vi "Handle Events.vi"(8 "error in (no error)":errorcluster, 11 "ListboxEventHandler":refnum<class "ListboxEventHandler.lvclass">) -> ()   [LabVIEW 2019, in "ActorEvents.lvlib" / "ListboxEventHandler.lvclass"]
uses:
  <vilib>/gpm_packages/@cs/mva-viewable/Source/ActorEvents/EventHandler/ListboxEventHandler/ListboxEventHandler.lvclass
  C:/Program Files/National Instruments/LabVIEW 2019/vi.lib/gpm_packages/@cs/mva-viewable/Source/ActorEvents/IEventHandler/IEventHandler.lvclass
  <vilib>/gpm_packages/@cs/mva-viewable/Source/ActorEvents/EventHandler/ListboxEventHandler/ListboxEventHandler.lvclass/ListboxEventHandler.ctl
  <vilib>/gpm_packages/@cs/mva-viewable/Source/ActorEvents/IEventHandler/IEventHandler.lvclass/IEventHandler.ctl
  <vilib>/ActorFramework/Message Enqueuer/Message Enqueuer.lvclass/Message Enqueuer.ctl
  <vilib>/event_ctls.llb/lveventtype.ctl
  <vilib>/gpm_packages/@cs/mva-viewable/Source/ActorEvents/IEventAggregator Messages/EventDataMessage/EventDataMessage.lvclass/EventDataMessage.ctl
  <vilib>/Utility/miscctls.llb/LVRowAndColumnTypeDef.ctl
  <vilib>/gpm_packages/@cs/mva-viewable/Source/ActorEvents/IEventAggregator Messages/ListboxEditCellMsg/ListboxEditCellMsg.lvclass/ListboxEditCellMsg.ctl
  <vilib>/gpm_packages/@cs/mva-viewable/Source/ActorEvents/IEventAggregator Messages/ControlKeyDownMsg/ControlKeyDownMsg.lvclass/ControlKeyDownMsg.ctl
  <vilib>/gpm_packages/@cs/mva-viewable/Source/ActorEvents/IEventAggregator Messages/ControlMouseDownMsg/ControlMouseDownMsg.lvclass/ControlMouseDownMsg.ctl
  <vilib>/gpm_packages/@cs/mva-viewable/Source/ActorEvents/IEventAggregator Messages/ControlDragStartingMsg/ControlDragStartingMsg.lvclass/ControlDragStartingMsg.ctl
  <vilib>/gpm_packages/@cs/mva-viewable/Source/ActorEvents/IEventAggregator Messages/ControlDragSourceUpdateMsg/ControlDragSourceUpdateMsg.lvclass/ControlDragSourceUpdateMsg.ctl
  <vilib>/gpm_packages/@cs/mva-viewable/Source/ActorEvents/IEventAggregator Messages/EventDataMessage/Read Discarded.vi
  <vilib>/gpm_packages/@cs/mva-viewable/Source/ActorEvents/IEventAggregator Messages/ListboxEditCellMsg/Accessors/Read String.vi
  <vilib>/gpm_packages/@cs/mva-viewable/Source/ActorEvents/IEventAggregator Messages/ControlKeyDownMsg/Accessors/Read Char.vi
  <vilib>/gpm_packages/@cs/mva-viewable/Source/ActorEvents/IEventAggregator Messages/ControlKeyDownMsg/Accessors/Read VKey.vi
  <vilib>/gpm_packages/@cs/mva-viewable/Source/ActorEvents/IEventAggregator Messages/ControlKeyDownMsg/Accessors/Read Mods.vi
  <vilib>/gpm_packages/@cs/mva-viewable/Source/ActorEvents/IEventAggregator Messages/ControlKeyDownMsg/Accessors/Read PlatMods.vi
  <vilib>/gpm_packages/@cs/mva-viewable/Source/ActorEvents/IEventAggregator Messages/ControlKeyDownMsg/Accessors/Read FocusObj.vi
  <vilib>/gpm_packages/@cs/mva-viewable/Source/ActorEvents/IEventAggregator Messages/ControlMouseDownMsg/Accessors/Read Button.vi
  <vilib>/gpm_packages/@cs/mva-viewable/Source/ActorEvents/IEventAggregator Messages/ControlMouseDownMsg/Accessors/Read Mods.vi
  <vilib>/gpm_packages/@cs/mva-viewable/Source/ActorEvents/IEventAggregator Messages/ControlMouseDownMsg/Accessors/Read PlatMods.vi
  <vilib>/gpm_packages/@cs/mva-viewable/Source/ActorEvents/IEventAggregator Messages/ControlDragStartingMsg/Accessors/Read Data.vi
  <vilib>/gpm_packages/@cs/mva-viewable/Source/ActorEvents/IEventAggregator Messages/ControlDragStartingMsg/Accessors/Read Drag Mode.vi
  <vilib>/gpm_packages/@cs/mva-viewable/Source/ActorEvents/IEventAggregator Messages/ControlDragSourceUpdateMsg/Accessors/Read Cursor.vi
  <vilib>/gpm_packages/@cs/mva-viewable/Source/ActorEvents/IEventHandler/Accessors/Read Timeout [ms].vi
  <vilib>/gpm_packages/@cs/mva-viewable/Source/ActorEvents/IEventHandler/Accessors/Read Event Filter.vi
  <vilib>/gpm_packages/@cs/mva-viewable/Source/ActorEvents/IEventHandler/Accessors/Read EventAggregator Enqueuer.vi
  <vilib>/gpm_packages/@cs/mva-viewable/Source/ActorEvents/IEventHandler/Accessors/Read Timeout Message.vi
  <vilib>/gpm_packages/@cs/mva-viewable/Source/ActorEvents/IEventHandler/Accessors/Read Timeout Message Priority.vi
  <vilib>/gpm_packages/@cs/mva-viewable/Source/ActorEvents/IEventAggregator Messages/ShortcutMenuSelectionMsg/ShortcutMenuSelectionMsg.lvclass
  C:/Program Files/National Instruments/LabVIEW 2019/vi.lib/gpm_packages/@cs/mva-viewable/Source/ActorEvents/IEventAggregator Messages/EventDataMessage/EventDataMessage.lvclass
  <vilib>/gpm_packages/@cs/mva-viewable/Source/ActorEvents/IEventAggregator Messages/ShortcutMenuActivationMsg/ShortcutMenuActivationMsg.lvclass
  <vilib>/gpm_packages/@cs/mva-viewable/Source/ActorEvents/IEventAggregator Messages/ListboxEditCellMsg/ListboxEditCellMsg.lvclass
  <vilib>/gpm_packages/@cs/mva-viewable/Source/ActorEvents/IEventAggregator Messages/ControlKeyDownMsg/ControlKeyDownMsg.lvclass
  <vilib>/gpm_packages/@cs/mva-viewable/Source/ActorEvents/IEventAggregator Messages/ControlMouseDownMsg/ControlMouseDownMsg.lvclass
  <vilib>/gpm_packages/@cs/mva-viewable/Source/ActorEvents/IEventAggregator Messages/ControlDropMsg/ControlDropMsg.lvclass
  <vilib>/gpm_packages/@cs/mva-viewable/Source/ActorEvents/IEventAggregator Messages/ControlDragOverMsg/ControlDragOverMsg.lvclass
  <vilib>/gpm_packages/@cs/mva-viewable/Source/ActorEvents/IEventAggregator Messages/ControlDragStartingMsg/ControlDragStartingMsg.lvclass
  <vilib>/gpm_packages/@cs/mva-viewable/Source/ActorEvents/IEventAggregator Messages/ControlDragSourceUpdateMsg/ControlDragSourceUpdateMsg.lvclass
  <vilib>/ActorFramework/Message Priority Queue/Priority Enqueue.vi
  <vilib>/gpm_packages/@cs/mva-viewable/Source/ActorEvents/IEventFilter/IEventFilter.lvclass
  <vilib>/ActorFramework/Message Enqueuer/Message Enqueuer.lvclass
  <vilib>/ActorFramework/Message/Message.lvclass
  <vilib>/gpm_packages/@cs/mva-viewable/Source/ActorEvents/IEventAggregator Messages/ValueChangeMsg/ValueChangeMsg.lvclass
  <vilib>/gpm_packages/@cs/mva-viewable/Source/ActorEvents/IEventAggregator Messages/ControlMouseUpMsg/ControlMouseUpMsg.lvclass
  <vilib>/gpm_packages/@cs/mva-viewable/Source/ActorEvents/IEventAggregator Messages/ListboxDoubleClickMsg/ListboxDoubleClickMsg.lvclass
  <vilib>/gpm_packages/@cs/mva-viewable/Source/ActorEvents/IEventAggregator Messages/ControlMouseEnterMsg/ControlMouseEnterMsg.lvclass
  <vilib>/gpm_packages/@cs/mva-viewable/Source/ActorEvents/IEventAggregator Messages/ControlMouseLeaveMsg/ControlMouseLeaveMsg.lvclass
  <vilib>/gpm_packages/@cs/mva-viewable/Source/ActorEvents/IEventAggregator Messages/ControlKeyUpMsg/ControlKeyUpMsg.lvclass
  <vilib>/gpm_packages/@cs/mva-viewable/Source/ActorEvents/IEventAggregator Messages/ControlDragEndedMsg/ControlDragEndedMsg.lvclass
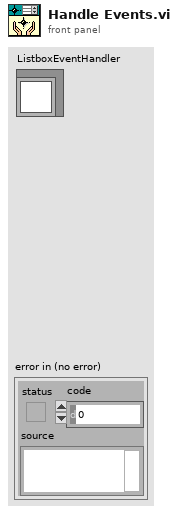
[diagram p1: front panel]
types:
  T1 = typedef "ActorEvents.lvlib/IEventFilter.lvclass/EventFilter Reference.ctl" = refnum<data-value>
  T2 = typedef "Actor Framework.lvlib/Message Enqueuer.lvclass/Message Priority.ctl" = enum16{"Low", "Normal", "High"}
  T3 = typedef "lveventtype.ctl" = enum32{"Null", "Timeout", "Annotation Menu Selection", "Annotation Menu Selection?", "App Instance Close", "App Instance Close?", "Autoscale Range Change", "Bookmark Info Change", "Cell Edit", "Cell Edit?", "Cursor Grab", "Cursor Grab?", "Cursor Menu Selection", "Cursor Menu Selection?", "Cursor Move", "Cursor Release", "Data Change", "Direction Change", "Display State Change", "Drag Ended", "Drag Enter", "Drag Leave", "Drag Over", "Drag Source Update", "Drag Starting", "Drag Starting?", "Drop", "Exec State Change", "Key Down", "Key Down?", "Key Repeat", "Key Repeat?", "Key Up", "Listbox Double Click", "Menu Activation?", "Menu Selection (App)", "Menu Selection? (App)", "Menu Selection (User)", "Mouse Down", "Mouse Down?", "Mouse Enter", "Mouse Leave", "Mouse Move", "Mouse Up", "Mouse Wheel", "NI Security User Change (App)", "Pane Size", "Panel Close", "Panel Close?", "Panel Resize", "Plot Attribute Change", "Scale Range Change", "Shortcut Menu Activation?", "Shortcut Menu Selection (App)", "Shortcut Menu Selection? (App)", "Shortcut Menu Selection (User)", "Tree Double Click", "Tree Drag", "Tree Drag?", "Tree Drop", "Tree Drop?", "Tree Item Close", "Tree Item Close?", "Tree Item Open", "Tree Item Open?", "User Event", "Value Change"}
  T4 = typedef "LVRowAndColumnTypeDef.ctl" = cluster{"Row":i32, "Column":i32}
  T5 = typedef "LVPoint32TypeDef.ctl" = cluster{"Horizontal":i32, "Vertical":i32}
  T6 = cluster{"Shift":bool, "Ctrl":bool, "Alt":bool, "Cmd":bool, "Opt":bool}
  T7 = typedef "eventvkey.ctl" = enum16{"ASCII", "Enter", "Return", "Shift", "Ctrl", "Alt", "Cmd", "Opt", "Caps", "NumLock", "Clear", "Break", "Up", "Down", "Left", "Right", "Insert", "Delete", "Home", "End", "PageUp", "PageDown", "Escape", "Help", "Pause", "ScrollLock", "F1", "F2", "F3", "F4", "F5", "F6", "F7", "F8", "F9", "F10", "F11", "F12", "F13", "F14", "F15", "F16", "F17", "F18", "F19", "F20", "F21", "F22", "F23", "F24", "Play", "VolumeUp", "VolumeDown", "Mute", "Two Byte Char"}
  T8 = cluster{"data name":string, "drag data":variant}[]
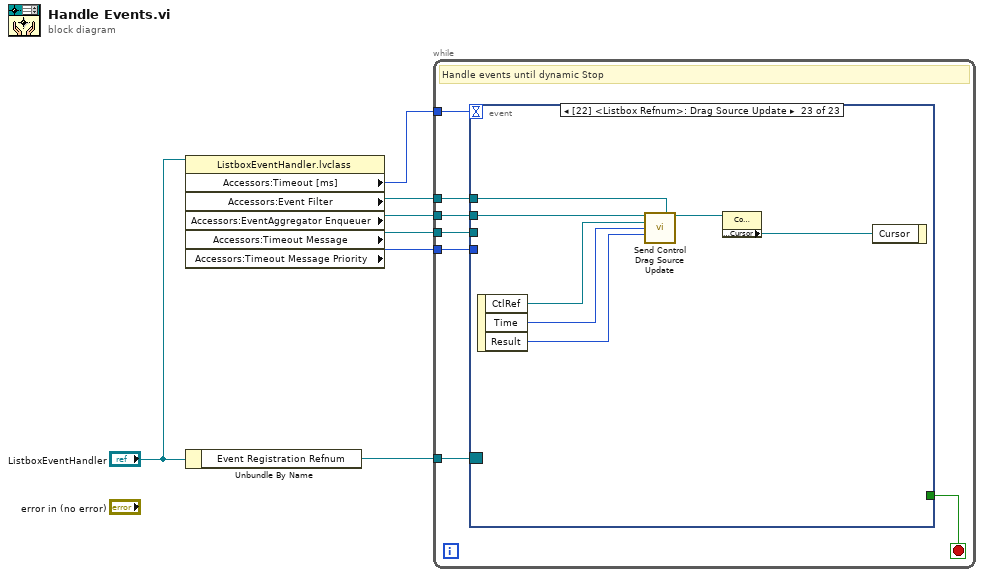
[diagram p0: block diagram]
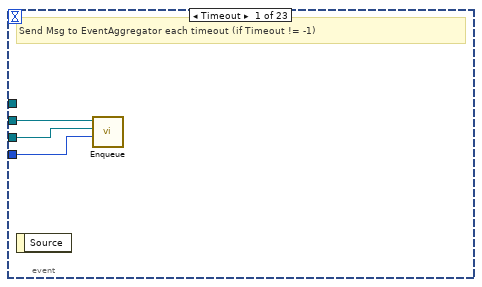
[diagram p2: hidden frame]
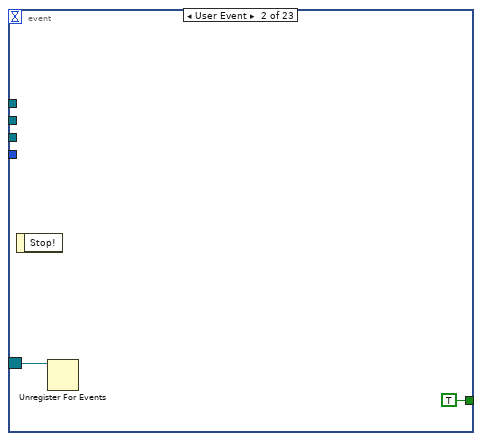
[diagram p3: hidden frame]
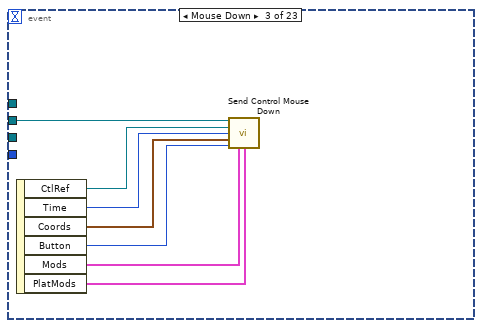
[diagram p4: hidden frame]
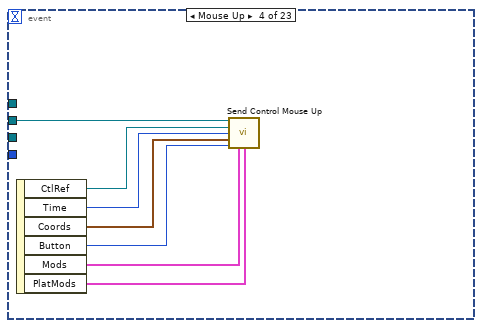
[diagram p5: hidden frame]
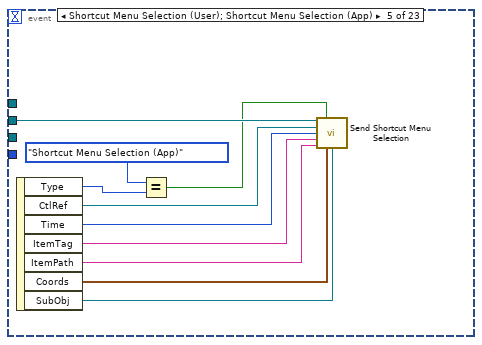
[diagram p6: hidden frame]
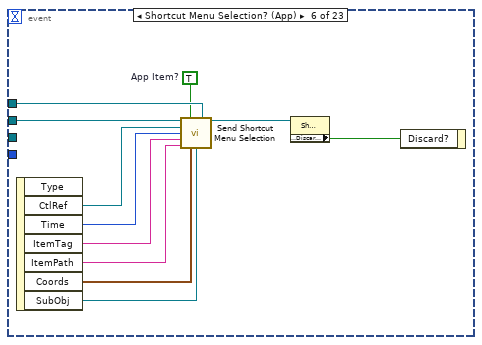
[diagram p7: hidden frame]
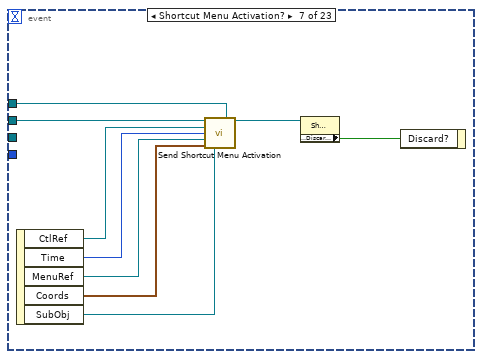
[diagram p8: hidden frame]
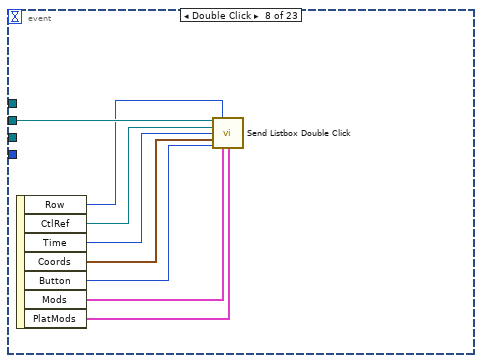
[diagram p9: hidden frame]
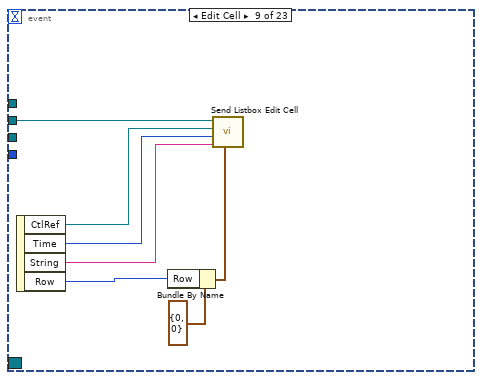
[diagram p10: hidden frame]
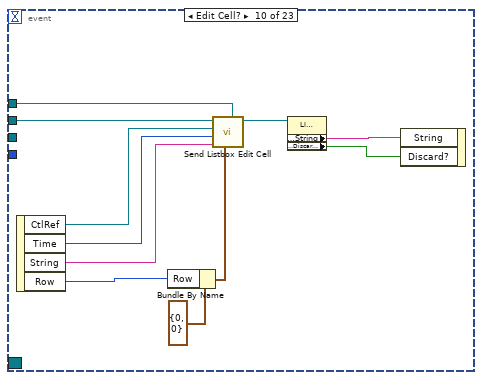
[diagram p11: hidden frame]
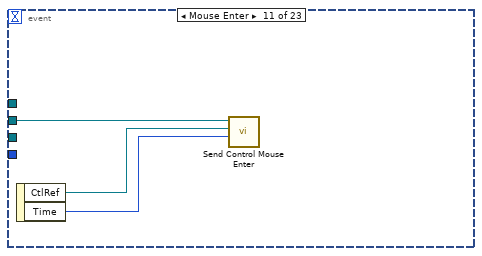
[diagram p12: hidden frame]
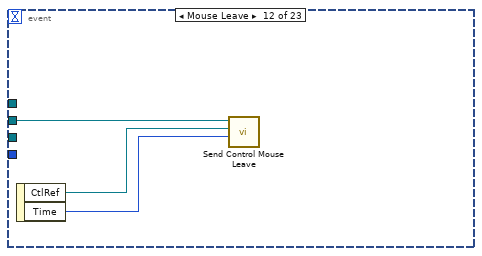
[diagram p13: hidden frame]
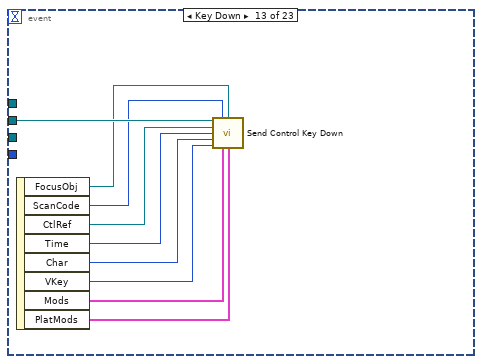
[diagram p14: hidden frame]
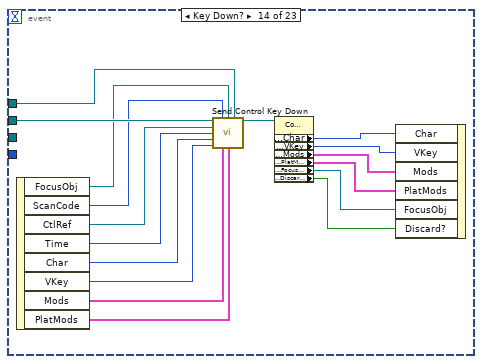
[diagram p15: hidden frame]
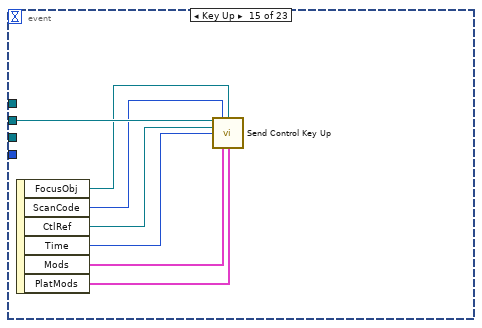
[diagram p16: hidden frame]
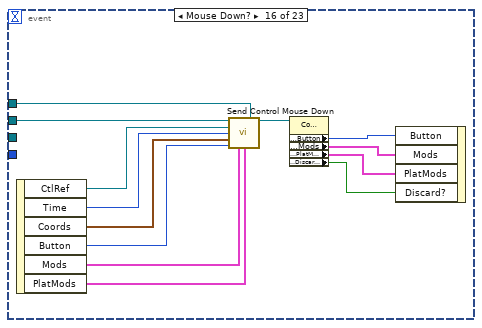
[diagram p17: hidden frame]
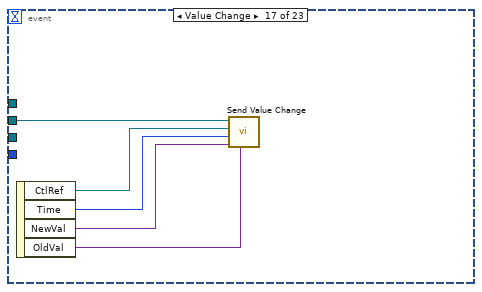
[diagram p18: hidden frame]
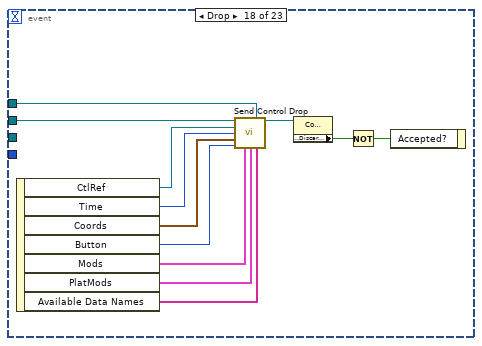
[diagram p19: hidden frame]
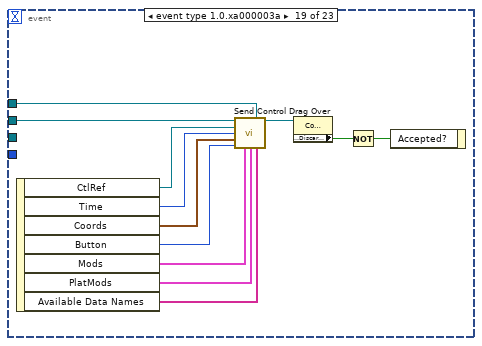
[diagram p20: hidden frame]
diagram:
  n1 = property class="ListboxEventHandler.lvclass"(reference="ListboxEventHandler") -> ("Accessors:Timeout [ms]"=w5:i32, "Accessors:Event Filter"=w3:T1, "Accessors:EventAggregator Enqueuer"=w4:refnum<class "Message Enqueuer.lvclass">, "Accessors:Timeout Message"=w2:refnum<class "Message.lvclass">, "Accessors:Timeout Message Priority"=w1:T2)  [unwired: 1 in, 2 out]
  n2 = Unbundle By Name("ListboxEventHandler") -> ("Event Registration Refnum"=w7:refnum<event-registration>)
  n3 = while {
    tunnel: w7 -> [w14]
    tunnel: w4 -> [w13]
    tunnel: w2 -> [w12]
    tunnel: w1 -> [w11]
    tunnel: w5 -> [w10]
    tunnel: w3 -> [w8]
    stop <- w9 stop-if-true
    # "Handle events until dynamic Stop"
    n4 = event shown="[22] <Listbox Refnum>: Drag Source Update" {
      selector: w14 -> [_ w19 _ _ _ _ _ _ _ _ _ _ _ _ _ _ _ _ _ _ _ _ _]
      dyn-events: _ -> [_ _ _ _ _ _ _ _ _ _ _ _ _ _ _ _ _ _ _ _ _ _ _]
      timeout: w10 -> [_ _ _ _ _ _ _ _ _ _ _ _ _ _ _ _ _ _ _ _ _ _ _]
      tunnel: [_ TRUE ("Stop!") _ _ _ _ _ _ _ _ _ _ _ _ _ _ _ _ _ _ _ _ _] -> w9
      tunnel: w13 -> [w17 _ w26 w33 w43 w54 w63 w71 w78 w89 w92 w95 w104 w121 w128 w141 w146 w156 w168 w174 w183 w197 w204]
      tunnel: w12 -> [w16 _ _ _ _ _ _ _ _ _ _ _ _ _ _ _ _ _ _ _ _ _ _]
      tunnel: w11 -> [w15 _ _ _ _ _ _ _ _ _ _ _ _ _ _ _ _ _ _ _ _ _ _]
      tunnel: w8 -> [_ _ _ _ _ w47 w57 _ _ w82 _ _ _ w111 _ w134 _ w147 w159 _ _ w187 w203]
      event Timeout {
        # "Send Msg to EventAggregator each timeout (if Timeout != -1)"
        n5 = event-data() -> ()  [unwired: 1 in, 1 out]
        n6 = call <vilib>:"Enqueue.vi"("Message Priority (Normal)"=w15, "Message"=w16, "Message Enqueuer in"=w17) -> ()  [unwired: 7 in, 2 out]
      }
      event User Event {
        n7 = event-data() -> ()  [unwired: 1 in, 1 out]
        n8 = Unregister For Events(event registration refnum=w19) -> ()  [unwired: 1 in, 1 out]
      }
      event Mouse Down {
        n9 = event-data() -> ("CtlRef"=w25:refnum<vi>, "Time"=w24:u32, "Coords"=w23:T5, "Button"=w22:u16, "Mods"=w21:cluster{"Double Click":bool, "Menu Key":bool}, "PlatMods"=w20:T6)  [unwired: 1 in]
        n10 = call <vilib>:"Send Control Mouse Down.vi"("Message Enqueuer in"=w26, "Ctl Refnum"=w25, "Time"=w24, "Coords"=w23, "Button"=w22, "Mods"=w21, "PlatMods"=w20) -> ()  [unwired: 7 in, 2 out]
      }
      event Mouse Up {
        n11 = event-data() -> ("CtlRef"=w32:refnum<vi>, "Time"=w31:u32, "Coords"=w30:T5, "Button"=w29:u16, "Mods"=w28:cluster{"Double Click":bool, "Menu Key":bool}, "PlatMods"=w27:T6)  [unwired: 1 in]
        n12 = call <vilib>:"Send Control Mouse Up.vi"("Message Enqueuer in"=w33, "Ctl Refnum"=w32, "Time"=w31, "Coords"=w30, "Button"=w29, "Mods"=w28, "PlatMods"=w27) -> ()  [unwired: 8 in, 1 out]
      }
      event Shortcut Menu Selection (User); Shortcut Menu Selection (App) {
        n13 = event-data() -> ("Type"=w36:T3, "CtlRef"=w42:refnum<vi>, "Time"=w41:u32, "ItemTag"=w40:string, "ItemPath"=w39:string, "Coords"=w38:T5, "SubObj"=w37:refnum<vi>)  [unwired: 1 in]
        n14 = Equal?(x=lveventtype."Shortcut Menu Selection (App)", y=w36) -> (x = y?=w35:bool)
        n15 = call <vilib>:"Send Shortcut Menu Selection.vi"("Message Enqueuer in"=w43, "App Item?"=w35, "CtlRef"=w42, "Time"=w41, "Item Tag"=w40, "Item Path"=w39, "Coords"=w38, "SubObj"=w37) -> ()  [unwired: 6 in, 2 out]
      }
      event Shortcut Menu Selection? (App) {
        w46 = TRUE  # App Item?
        n16 = event-data() -> ("CtlRef"=w53:refnum<vi>, "Time"=w52:u32, "ItemTag"=w51:string, "ItemPath"=w50:string, "Coords"=w49:T5, "SubObj"=w48:refnum<vi>)  [unwired: 1 in, 1 out]
        n17 = call <vilib>:"Send Shortcut Menu Selection.vi"("Message Enqueuer in"=w54, "App Item?"=w46, "EventFilter Reference"=w47, "CtlRef"=w53, "Time"=w52, "Item Tag"=w51, "Item Path"=w50, "Coords"=w49, "SubObj"=w48) -> ("Filtered EventDataMessage"=w45:refnum<class "ShortcutMenuSelectionMsg.lvclass">)  [unwired: 5 in, 1 out]
        n18 = property class="ShortcutMenuSelectionMsg.lvclas"(reference=w45) -> ("Accessors:Discarded?"=w44:bool)  [unwired: 1 in, 2 out]
        n19 = event-data("Discard?"=w44) -> ()  [unwired: 1 in, 1 out]
      }
      event Shortcut Menu Activation? {
        n20 = event-data() -> ("CtlRef"=w58:refnum<vi>, "Time"=w62:u32, "MenuRef"=w59:refnum<k9>, "Coords"=w61:T5, "SubObj"=w60:refnum<vi>)  [unwired: 1 in]
        n21 = call <vilib>:"Send Shortcut Menu Activation.vi"("Message Enqueuer in"=w63, "EventFilter Reference"=w57, "CtlRef"=w58, "Time"=w62, "MenuRef"=w59, "Coords"=w61, "SubObj"=w60) -> ("Filtered EventDataMessage"=w56:refnum<class "ShortcutMenuActivationMsg.lvclass">)  [unwired: 7 in, 1 out]
        n22 = property class="ShortcutMenuActivationMsg.lvcla"(reference=w56) -> ("Accessors:Discarded?"=w55:bool)  [unwired: 1 in, 2 out]
        n23 = event-data("Discard?"=w55) -> ()  [unwired: 1 in, 1 out]
      }
      event Double Click {
        n24 = event-data() -> ("Row"=w64:i32, "CtlRef"=w70:refnum<vi>, "Time"=w69:u32, "Coords"=w68:T5, "Button"=w67:u16, "Mods"=w66:cluster{"Double Click":bool, "Menu Key":bool}, "PlatMods"=w65:T6)  [unwired: 1 in]
        n25 = call <vilib>:"Send Listbox Double Click.vi"("Message Enqueuer in"=w71, "Row"=w64, "Ctl Refnum"=w70, "Time"=w69, "Coords"=w68, "Button"=w67, "Mods"=w66, "PlatMods"=w65) -> ()  [unwired: 7 in, 1 out]
      }
      event Edit Cell {
        n26 = event-data() -> ("CtlRef"=w77:refnum<vi>, "Time"=w76:u32, "String"=w75:string, "Row"=w74:i32)  [unwired: 1 in]
        n27 = Bundle By Name(cluster=T4 {"Row"=0, "Column"=0} ("Coords"), "Row"=w74) -> (w72:T4)
        n28 = call <vilib>:"Send Listbox Edit Cell.vi"("Coords"=w72, "String"=w75, "Time"=w76, "CtlRef"=w77, "Message Enqueuer in"=w78) -> ()  [unwired: 5 in, 2 out]
      }
      event Edit Cell? {
        n29 = event-data() -> ("CtlRef"=w88:refnum<vi>, "Time"=w87:u32, "String"=w86:string, "Row"=w85:i32)  [unwired: 1 in]
        n30 = Bundle By Name(cluster=T4 {"Row"=0, "Column"=0} ("Coords"), "Row"=w85) -> (w83:T4)
        n31 = call <vilib>:"Send Listbox Edit Cell.vi"("EventFilter Reference"=w82, "Coords"=w83, "String"=w86, "Time"=w87, "CtlRef"=w88, "Message Enqueuer in"=w89) -> ("Filtered EventDataMessage"=w81:refnum<class "ListboxEditCellMsg.lvclass">)  [unwired: 4 in, 1 out]
        n32 = property class="ListboxEditCellMsg.lvclass"(reference=w81) -> ("Accessors:String"=w80:string, "Accessors:Discarded?"=w79:bool)  [unwired: 1 in, 2 out]
        n33 = event-data("String"=w80, "Discard?"=w79) -> ()  [unwired: 1 in, 1 out]
      }
      event Mouse Enter {
        n34 = event-data() -> ("CtlRef"=w91:refnum<vi>, "Time"=w90:u32)  [unwired: 1 in]
        n35 = call <vilib>:"Send Control Mouse Enter.vi"("Time"=w90, "Ctl Refnum"=w91, "Message Enqueuer in"=w92) -> ()  [unwired: 8 in, 1 out]
      }
      event Mouse Leave {
        n36 = event-data() -> ("CtlRef"=w94:refnum<vi>, "Time"=w93:u32)  [unwired: 1 in]
        n37 = call <vilib>:"Send Control Mouse Leave.vi"("Time"=w93, "Ctl Refnum"=w94, "Message Enqueuer in"=w95) -> ()  [unwired: 8 in, 1 out]
      }
      event Key Down {
        n38 = event-data() -> ("FocusObj"=w103:refnum<vi>, "ScanCode"=w102:i16, "CtlRef"=w101:refnum<vi>, "Time"=w100:u32, "Char"=w99:i16, "VKey"=w98:T7, "Mods"=w97:cluster{"Num Pad":bool, "Menu Key":bool}, "PlatMods"=w96:T6)  [unwired: 1 in]
        n39 = call <vilib>:"Send Control Key Down.vi"("Message Enqueuer in"=w104, "ScanCode"=w102, "FocusObj"=w103, "CtlRef"=w101, "Time"=w100, "Char"=w99, "VKey"=w98, "Mods"=w97, "PlatMods"=w96) -> ()  [unwired: 5 in, 2 out]
      }
      event Key Down? {
        n40 = event-data() -> ("FocusObj"=w120:refnum<vi>, "ScanCode"=w119:i16, "CtlRef"=w118:refnum<vi>, "Time"=w117:u32, "Char"=w116:i16, "VKey"=w115:T7, "Mods"=w114:cluster{"Num Pad":bool, "Menu Key":bool}, "PlatMods"=w113:T6)  [unwired: 1 in]
        n41 = call <vilib>:"Send Control Key Down.vi"("Message Enqueuer in"=w121, "ScanCode"=w119, "FocusObj"=w120, "EventFilter Reference"=w111, "CtlRef"=w118, "Time"=w117, "Char"=w116, "VKey"=w115, "Mods"=w114, "PlatMods"=w113) -> ("Filtered EventDataMessage"=w112:refnum<class "ControlKeyDownMsg.lvclass">)  [unwired: 4 in, 1 out]
        n42 = property class="ControlKeyDownMsg.lvclass"(reference=w112) -> ("Accessors:Char"=w110:i16, "Accessors:VKey"=w109:T7, "Accessors:Mods"=w108:cluster{"Double Click":bool, "Menu Key":bool}, "Accessors:PlatMods"=w107:T6, "Accessors:FocusObj"=w106:refnum<vi>, "Accessors:Discarded?"=w105:bool)  [unwired: 1 in, 2 out]
        n43 = event-data("Char"=w110, "VKey"=w109, "Mods"=w108, "PlatMods"=w107, "FocusObj"=w106, "Discard?"=w105) -> ()  [unwired: 1 in, 1 out]
      }
      event Key Up {
        n44 = event-data() -> ("FocusObj"=w127:refnum<vi>, "ScanCode"=w126:i16, "CtlRef"=w125:refnum<vi>, "Time"=w124:u32, "Mods"=w123:cluster{"Num Pad":bool, "Menu Key":bool}, "PlatMods"=w122:T6)  [unwired: 1 in]
        n45 = call <vilib>:"Send Control Key Up.vi"("Message Enqueuer in"=w128, "ScanCode"=w126, "FocusObj"=w127, "Ctl Refnum"=w125, "Time"=w124, "Mods"=w123, "PlatMods"=w122) -> ()  [unwired: 8 in, 1 out]
      }
      event Mouse Down? {
        n46 = event-data() -> ("CtlRef"=w140:refnum<vi>, "Time"=w139:u32, "Coords"=w138:T5, "Button"=w137:u16, "Mods"=w136:cluster{"Double Click":bool, "Menu Key":bool}, "PlatMods"=w135:T6)  [unwired: 1 in]
        n47 = call <vilib>:"Send Control Mouse Down.vi"("Message Enqueuer in"=w141, "EventFilter Reference"=w134, "Ctl Refnum"=w140, "Time"=w139, "Coords"=w138, "Button"=w137, "Mods"=w136, "PlatMods"=w135) -> ("Filtered EventDataMessage"=w133:refnum<class "ControlMouseDownMsg.lvclass">)  [unwired: 6 in, 1 out]
        n48 = property class="ControlMouseDownMsg.lvclass"(reference=w133) -> ("Accessors:Button"=w132:u16, "Accessors:Mods"=w131:cluster{"Double Click":bool, "Menu Key":bool}, "Accessors:PlatMods"=w130:T6, "Accessors:Discarded?"=w129:bool)  [unwired: 1 in, 2 out]
        n49 = event-data("Button"=w132, "Mods"=w131, "PlatMods"=w130, "Discard?"=w129) -> ()  [unwired: 1 in, 1 out]
      }
      event Value Change {
        n50 = event-data() -> ("CtlRef"=w143:refnum<vi>, "Time"=w145:u32, "NewVal"=w144:variant, "OldVal"=w142:variant)  [unwired: 1 in]
        n51 = call <vilib>:"Send Value Change.vi"("Old Value"=w142, "New Value"=w144, "Time"=w145, "Ctl Refnum"=w143, "Message Enqueuer in"=w146) -> ()  [unwired: 6 in, 1 out]
      }
      event Drop {
        n52 = event-data() -> ("CtlRef"=w154:refnum<vi>, "Time"=w153:u32, "Coords"=w152:T5, "Button"=w151:u16, "Mods"=w150:cluster{"Double Click":bool, "Menu Key":bool}, "PlatMods"=w149:T6, "Available Data Names"=w148:string[])  [unwired: 1 in]
        n53 = call <vilib>:"Send Control Drop.vi"("Message Enqueuer in"=w156, "EventFilter Reference"=w147, "CtlRef"=w154, "Time"=w153, "Coords"=w152, "Button"=w151, "Mods"=w150, "PlatMods"=w149, "Available Data Names"=w148) -> ("Filtered EventDataMessage"=w157:refnum<class "ControlDropMsg.lvclass">)  [unwired: 5 in, 1 out]
        n54 = property class="ControlDropMsg.lvclass"(reference=w157) -> ("Accessors:Discarded?"=w158:bool)  [unwired: 1 in, 2 out]
        n55 = Not(x=w158) -> (.not. x?=w155:bool)
        n56 = event-data("Accepted?"=w155) -> ()  [unwired: 1 in, 1 out]
      }
      event event type 1.0.xa000003a {
        n57 = event-data() -> ("CtlRef"=w166:refnum<vi>, "Time"=w165:u32, "Coords"=w164:T5, "Button"=w163:u16, "Mods"=w162:cluster{"Double Click":bool, "Menu Key":bool}, "PlatMods"=w161:T6, "Available Data Names"=w160:string[])  [unwired: 1 in]
        n58 = call <vilib>:"Send Control Drag Over.vi"("Message Enqueuer in"=w168, "EventFilter Reference"=w159, "CtlRef"=w166, "Time"=w165, "Coords"=w164, "Button"=w163, "Mods"=w162, "PlatMods"=w161, "Available Data Names"=w160) -> ("Filtered EventDataMessage"=w169:refnum<class "ControlDragOverMsg.lvclass">)  [unwired: 5 in, 1 out]
        n59 = property class="ControlDragOverMsg.lvclass"(reference=w169) -> ("Accessors:Discarded?"=w170:bool)  [unwired: 1 in, 2 out]
        n60 = Not(x=w170) -> (.not. x?=w167:bool)
        n61 = event-data("Accepted?"=w167) -> ()  [unwired: 1 in, 1 out]
      }
      event Drag Ended {
        n62 = event-data() -> ("CtlRef"=w173:refnum<vi>, "Time"=w172:u32, "Result"=w171:enum16{"Drop Cancel", "Drop Move", "Drop Copy"})  [unwired: 1 in]
        n63 = call <vilib>:"Send Control Drag Ended.vi"("Message Enqueuer in"=w174, "CtlRef"=w173, "Time"=w172, "Result"=w171) -> ()  [unwired: 10 in, 2 out]
      }
      event Drag Starting {
        n64 = event-data() -> ("Drag Mode"=w182:enum32{"copy or move", "copy only", "move only"}, "CtlRef"=w181:refnum<vi>, "Time"=w180:u32, "Coords"=w179:T5, "Button"=w178:u16, "Mods"=w177:cluster{"Double Click":bool, "Menu Key":bool}, "PlatMods"=w176:T6, "Data"=w175:T8)  [unwired: 1 in]
        n65 = call <vilib>:"Send Control Drag Starting.vi"("Message Enqueuer in"=w183, "Drag Mode"=w182, "CtlRef"=w181, "Time"=w180, "Coords"=w179, "Button"=w178, "Mods"=w177, "PlatMods"=w176, "Data"=w175) -> ()  [unwired: 5 in, 2 out]
      }
      event Drag Starting? {
        n66 = event-data() -> ("Drag Mode"=w196:enum32{"copy or move", "copy only", "move only"}, "CtlRef"=w195:refnum<vi>, "Time"=w194:u32, "Coords"=w193:T5, "Button"=w192:u16, "Mods"=w191:cluster{"Double Click":bool, "Menu Key":bool}, "PlatMods"=w190:T6, "Data"=w189:T8)  [unwired: 1 in]
        n67 = call <vilib>:"Send Control Drag Starting.vi"("Message Enqueuer in"=w197, "Drag Mode"=w196, "EventFilter Reference"=w187, "CtlRef"=w195, "Time"=w194, "Coords"=w193, "Button"=w192, "Mods"=w191, "PlatMods"=w190, "Data"=w189) -> ("Filtered EventDataMessage"=w188:refnum<class "ControlDragStartingMsg.lvclass">)  [unwired: 4 in, 1 out]
        n68 = property class="ControlDragStartingMsg.lvclass"(reference=w188) -> ("Accessors:Data"=w186:T8, "Accessors:Drag Mode"=w185:enum32{"copy or move", "copy only", "move only"}, "Accessors:Discarded?"=w184:bool)  [unwired: 1 in, 2 out]
        n69 = event-data("Data"=w186, "Drag Mode"=w185, "Discard?"=w184) -> ()  [unwired: 1 in, 1 out]
      }
      event Drag Source Update {
        n70 = event-data() -> ("CtlRef"=w202:refnum<vi>, "Time"=w201:u32, "Result"=w200:enum16{"Drop Cancel", "Drop Move", "Drop Copy"})  [unwired: 1 in]
        n71 = call <vilib>:"Send Control Drag Source Update.vi"("Message Enqueuer in"=w204, "EventFilter Reference"=w203, "CtlRef"=w202, "Time"=w201, "Result"=w200) -> ("Filtered EventDataMessage"=w199:refnum<class "ControlDragSourceUpdateMsg.lvclass">)  [unwired: 9 in, 1 out]
        n72 = property class="ControlDragSourceUpdateMsg.lvcl"(reference=w199) -> ("Accessors:Cursor"=w198:refnum<k1>)  [unwired: 1 in, 2 out]
        n73 = event-data("Cursor"=w198) -> ()  [unwired: 1 in, 1 out]
      }
    }
  }
